vi "Periodic Tasks.vi"(8 "error in":errorcluster) -> ()   [LabVIEW 2020]
doc: "This VI runs in parallel to other tasks. It can contain as many user-defined periodic loops as you need. These can carry out PID or other sorts of timed response."
uses:
  <vilib>/Rock Robotics/WPI/ThirdParty/Sensors/navX/_TypeDefs/FRIC_navX_DeviceNumbersTypeDef.ctl
  <vilib>/Rock Robotics/WPI/ThirdParty/REV Robotics/REVLib/Typedef/Spark MAX Control Type.ctl
  <vilib>/Rock Robotics/WPI/ThirdParty/JAS_Junk/TrajLib/Rotation2d_CreateAngle.vi
  Robot Global Data.vi
  <vilib>/Rock Robotics/Network Tables/NT Write Boolean.vi
  <vilib>/Rock Robotics/Network Tables/NT Write Number.vi
  <vilib>/Rock Robotics/WPI/ThirdParty/Phoenix-LabVIEW/CANCoder/Get/CTRE_Phoenix_CANcoder_GetSensorData.vi
  Dawgma Programming Library/Utilities/armSetpoints.vi
  <vilib>/addons/control/pid/pid.llb/PID (DBL).vi
  <vilib>/Rock Robotics/WPI/ThirdParty/JAS_Junk/TrajLib/Trajectory_Library.lvlib
  <vilib>/addons/control/pid/NI_PID_pid.lvlib
  <vilib>/Rock Robotics/Network Tables/NT Read Boolean.vi
panel:
  out "arm position":dbl=0.11904771625995636
  out "Sensor Position":dbl=-2.8186375402583508e-06
  out "output":dbl=1.265315424634228e-06 format="%.2f"
  in  "SPOOL PID":T1={"proportional gain (Kc)"=0.44891030029999945, "integral time (Ti, min)"=0.0, "derivative time (Td, min)"=0.0} {"derivative time (Td, min)" format="%.29f"; "integral time (Ti, min)" format="%.29f"; "proportional gain (Kc)" format="%.29f"}
  out "arm output":dbl=0.02326189109385013 format="%.2f"
  in  "FeedFwd Value":dbl=0.04 format="%.2f"
  in  "ARM PID":T1={"proportional gain (Kc)"=0.14060000000000006, "integral time (Ti, min)"=0.0, "derivative time (Td, min)"=0.0} {"derivative time (Td, min)" format="%.15f"; "integral time (Ti, min)" format="%.15f"; "proportional gain (Kc)" format="%.15f"}
  out "POSE.TRANSLATION.Y":dbl=0.0014854368037226463
  out "POSE.TRANSLATION.X":dbl=0.0024920325622980453
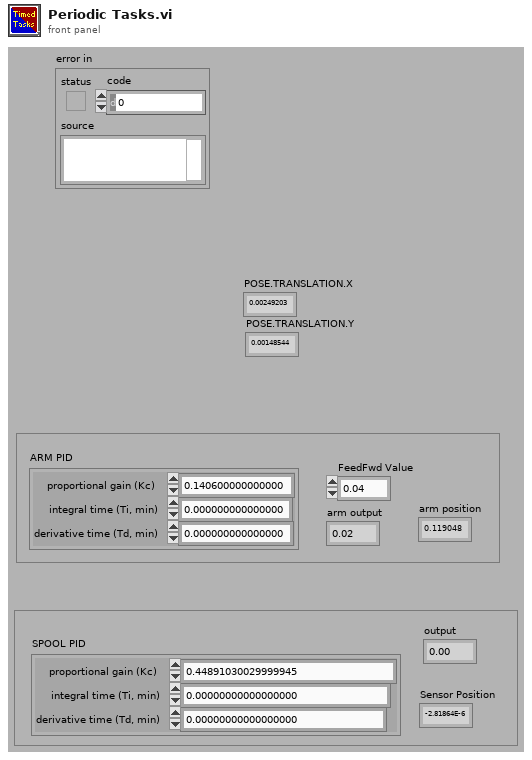
[diagram p1: front panel]
types:
  T1 = cluster{"proportional gain (Kc)":dbl, "integral time (Ti, min)":dbl, "derivative time (Td, min)":dbl}
  T2 = typedef "Trajectory_Library.lvlib/ROTATION2D.ctl" = cluster{"VALUE":dbl, "COS":dbl, "SIN":dbl}
  T3 = typedef "Trajectory_Library.lvlib/TRANSLATION2D.ctl" = cluster{"X":dbl, "Y":dbl}
  T4 = typedef "Trajectory_Library.lvlib/SWERVE_DRIVE_MODULE_POSITION.ctl" = cluster{"Distance":dbl, "Angle":T2, "P":bool}
  T5 = typedef "Trajectory_Library.lvlib/POSE2D.ctl" = cluster{"TRANSLATION":T3, "ROTATION":T2}
  T6 = typedef "Trajectory_Library.lvlib/SWERVE_DRIVE_KINEMATICS.ctl" = cluster{"NumModules":i32, "InverseKinematics":T7, "ForwardKinematics":T7, "Modules":T3[], "PrevCoR":T3, "SavedModuleStates":T8[]}
  T7 = typedef "NI_Matrix.lvlib/RealMatrix.ctl" = dbl[][]
  T8 = typedef "Trajectory_Library.lvlib/SWERVE_DRIVE_MODULE_STATE.ctl" = cluster{"Speed":dbl, "Angle":T2}
  T9 = typedef "Trajectory_Library.lvlib/SWERVE_DRIVE_ODOMETRY.ctl" = cluster{"POSE":T5, "GyroOffset":T2, "PreviousAngle":T2, "PrevModulePositions":T4[], "NumModules":i32}
  T10 = typedef "WPI_MotorControlDeviceRef.ctl" = cluster{"DeviceStatus":errorcluster, "Type":T11, "PWM":cluster{"PWM Channel":T12, "DeadBand":T13}, "CAN":cluster{"Device Number":u8, "SetOutput VI Ref":variant, "GetOutput VI Ref":variant, "Enable VI Ref":variant, "Disable VI Ref":variant, "Data":variant}, "Invert":bool, "DIO PWM":cluster{"PWM \"Enable\" Channel":T12, "DIOChannel":T14, "PWM Rate":dbl}}
  T11 = typedef "WPI_MotorControlType.ctl" = enum16{"PWM", "CAN", "DIO PWM"}
  T12 = typedef "FPGA_DIOPWMChannel.ctl" = enum8{"PWM 0", "PWM 1", "PWM 2", "PWM 3", "PWM 4", "PWM 5", "PWM 6", "PWM 7", "PWM 8", "PWM 9", "PWM MXP 0", "PWM MXP 1", "PWM MXP 2", "PWM MXP 3", "PWM MXP 4", "PWM MXP 5", "PWM MXP 6", "PWM MXP 7", "PWM MXP 8", "PWM MXP 9", "Invalid"}
  T13 = typedef "WPI_PWMDeadband.ctl" = cluster{"Name":string, "maxPositivePwm":i32, "minPositivePwm":i32, "centerPwm":i32, "maxNegativePwm":i32, "minNegativePwm":i32, "angularRange":u16}
  T14 = typedef "FPGA_DIOChannel.ctl" = enum8{"DIO 0", "DIO 1", "DIO 2", "DIO 3", "DIO 4", "DIO 5", "DIO 6", "DIO 7", "DIO 8", "DIO 9", "DIO MXP 0", "DIO MXP 1", "DIO MXP 2", "DIO MXP 3", "DIO MXP 4", "DIO MXP 5", "DIO MXP 6", "DIO MXP 7", "DIO MXP 8", "DIO MXP 9", "DIO MXP 10", "DIO MXP 11", "DIO MXP 12", "DIO MXP 13", "DIO MXP 14", "DIO MXP 15", "SPI Port CS1", "SPI Port CS2", "SPI Port CS3", "SPI Port MISO", "SPI Port MOSI", "Invalid"}
  T15 = typedef "FRIC_navX_DeviceNumbersTypeDef.ctl" = enum16{"Dev0", "Dev1", "Dev2", "Dev3"}
  T16 = cluster{"POSE.TRANSLATION.X":dbl, "POSE.TRANSLATION.Y":dbl}
  T17 = typedef "Spark MAX Control Type.ctl" = enum16{"Percent VBus", "Voltage", "Velocity", "Position", "Smart Motion", "Current", "Smart Velocity"}
  T18 = cluster{"Yaw":dbl, "Roll":dbl, "Pitch":dbl, "Heading":dbl, "Fused Heading":dbl}
  T19 = cluster{"Arm pos":dbl, "Sensor Position":dbl, "Spool pos":dbl, "Sensor Position":dbl}
  T20 = typedef "CTRE_Phoenix_CANcoder_DeviceRef.ctl" = cluster{"DeviceStatus":errorcluster, "Device Number":u8, "Handle":u64, "UsageFrame":u32, "Library Path":path}
  T21 = cluster{"FL":cluster{"proportional gain (Kc)":dbl, "integral time (Ti, min)":dbl, "derivative time (Td, min)":dbl}, "FR":cluster{"proportional gain (Kc)":dbl, "integral time (Ti, min)":dbl, "derivative time (Td, min)":dbl}, "BL":cluster{"proportional gain (Kc)":dbl, "integral time (Ti, min)":dbl, "derivative time (Td, min)":dbl}, "BR":cluster{"proportional gain (Kc)":dbl, "integral time (Ti, min)":dbl, "derivative time (Td, min)":dbl}}
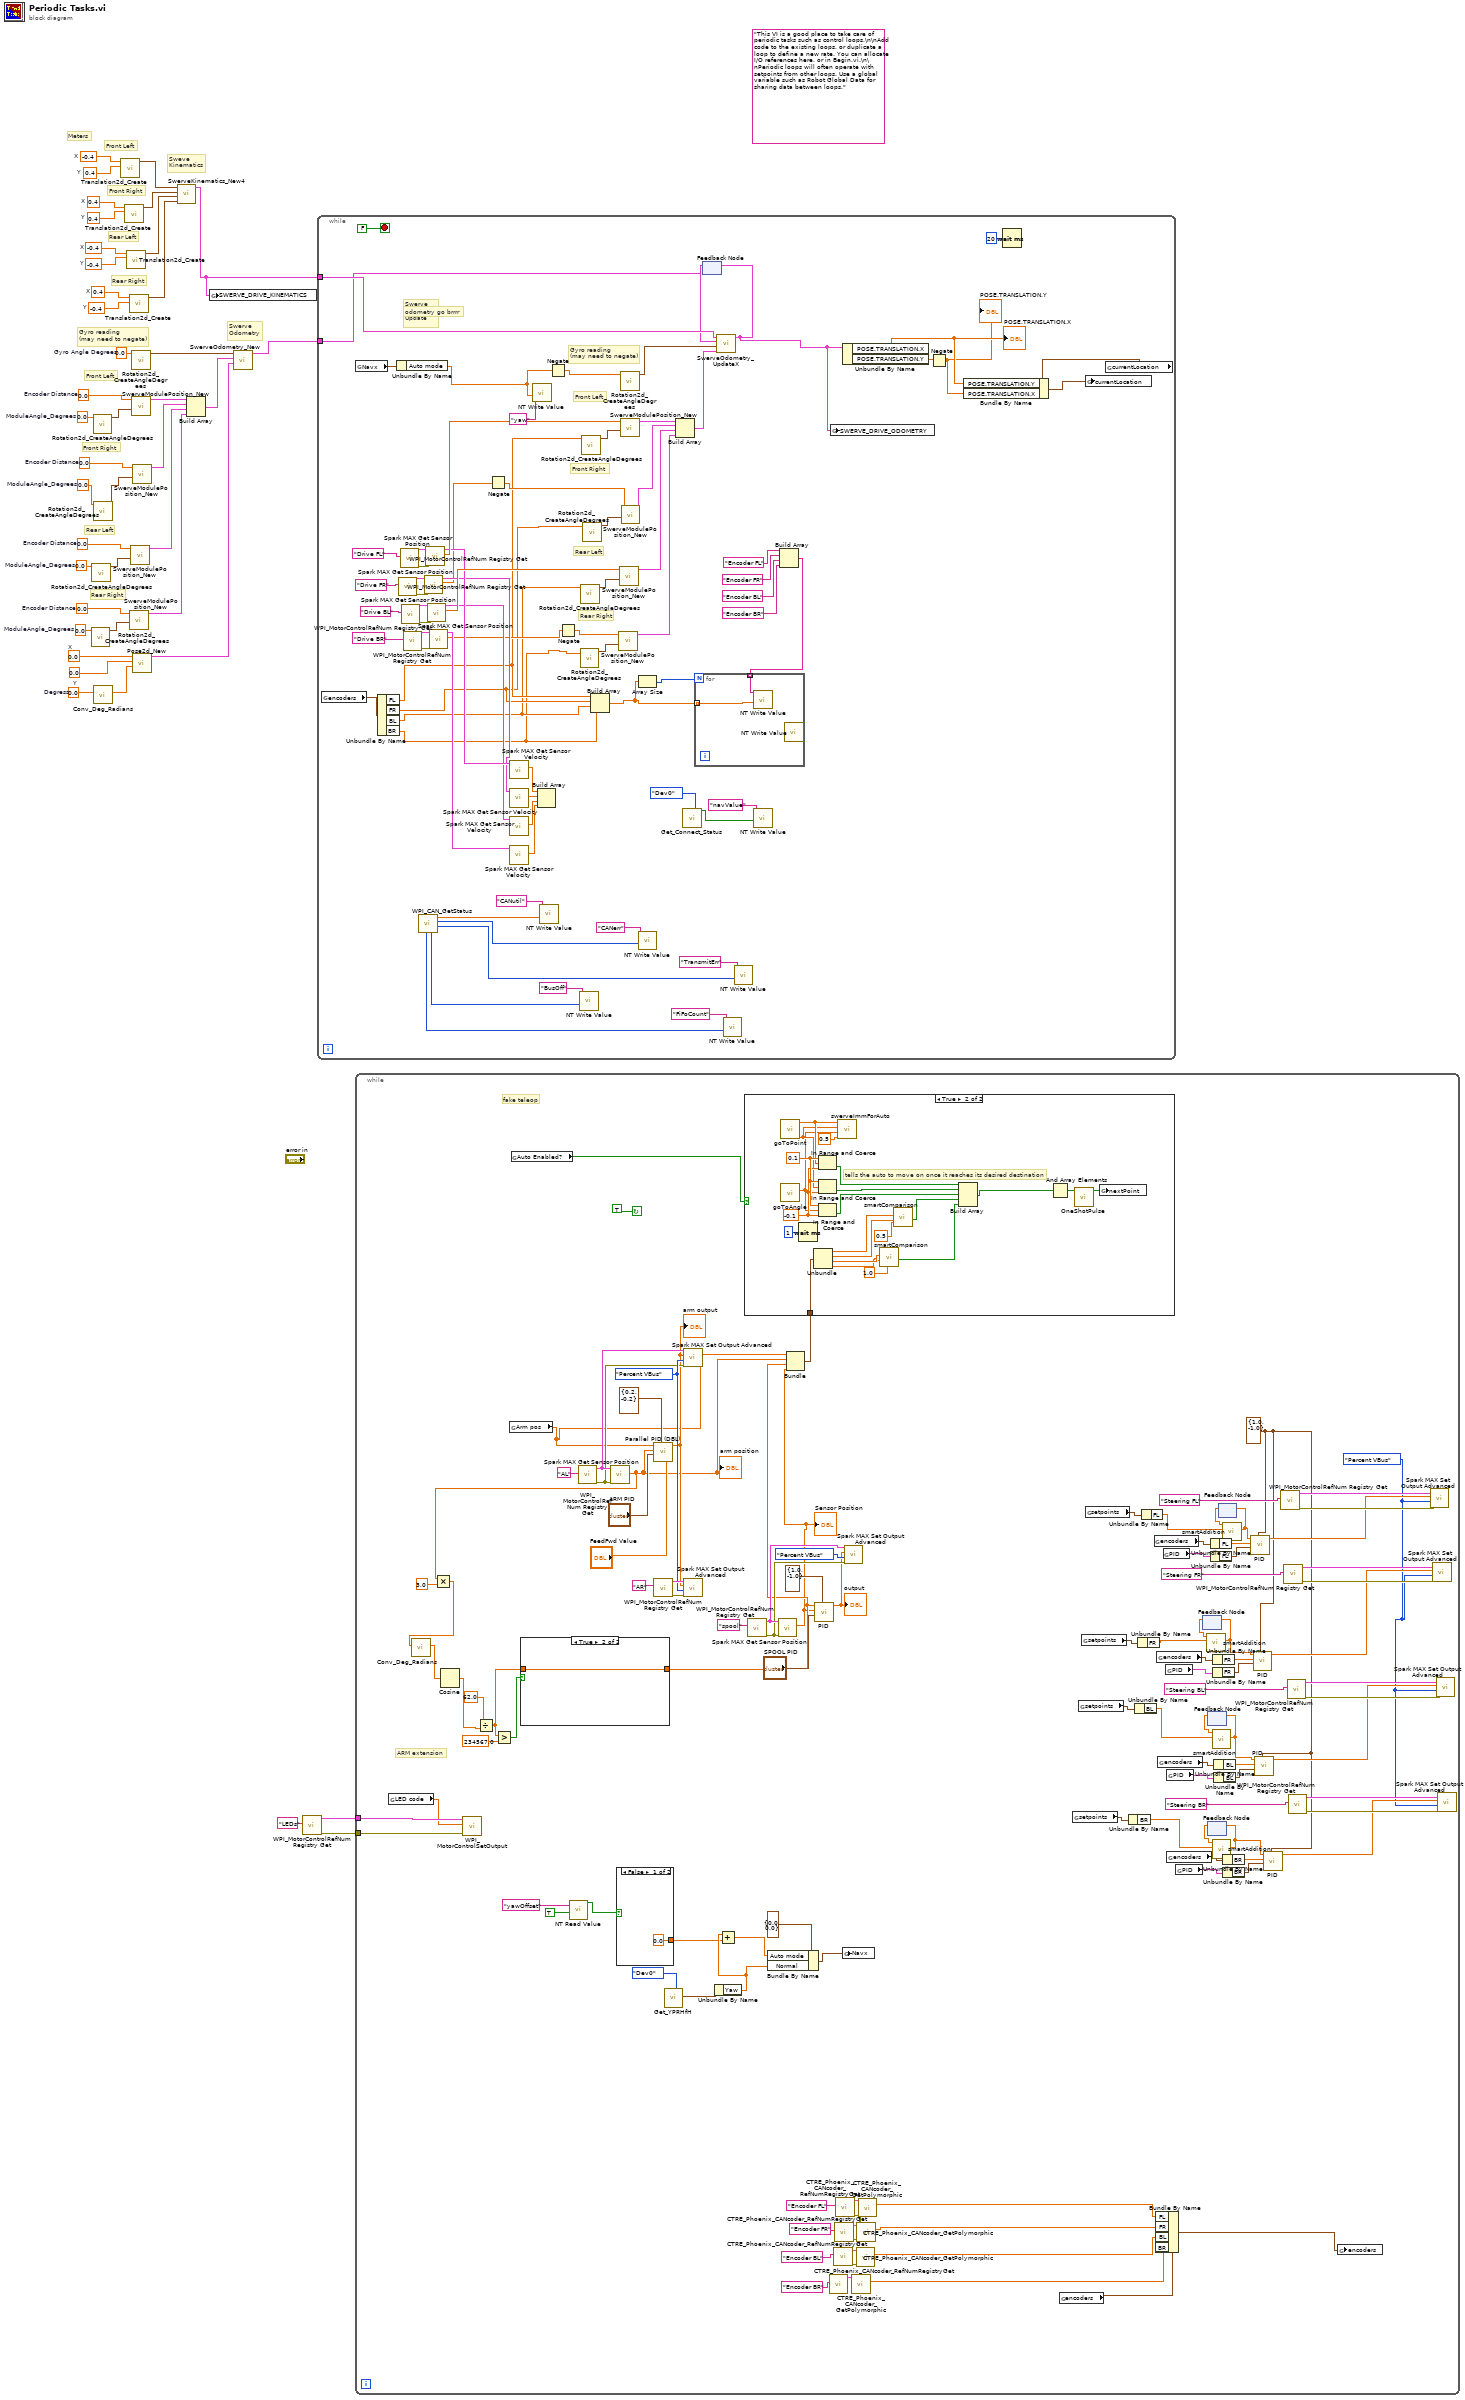
[diagram p0: block diagram]
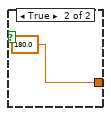
[diagram p2: hidden frame]
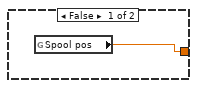
[diagram p3: hidden frame]
diagram:
  w12 = 0.4  # X
  w11 = -0.4  # Y
  w10 = -0.4  # X
  w9 = -0.4  # Y
  w8 = 0.4  # X
  w7 = 0.4  # Y
  w6 = -0.4  # X
  w5 = 0.4  # Y
  w40 = 0.0  # Degress
  w39 = 0.0  # X
  w38 = 0.0  # Y
  w31 = 0.0  # ModuleAngle_Degrees
  w29 = 0.0  # Encoder Distance
  w28 = 0.0  # ModuleAngle_Degrees
  w26 = 0.0  # Encoder Distance
  w25 = 0.0  # ModuleAngle_Degrees
  w23 = 0.0  # Encoder Distance
  w21 = 0.0  # Gyro Angle Degrees
  w20 = 0.0  # ModuleAngle_Degrees
  w18 = 0.0  # Encoder Distance
  (unwired) "This VI is a good place to take care of periodic tasks such as control loops.\n\nAdd code to the existing loops, or duplicate a loop to define a new rate. You can allocate I/O references here, or in Begin.vi.\n\nPeriodic loops will often operate with setpoints from other loops. Use a global variable such as Robot Global Data for sharing data between loops."
  # "Meters"
  # "Sweve\nKinematics"
  # "Rear Right"
  # "Rear Left"
  # "Front Right"
  # "Front Left"
  # "Swerve\nOdometry"
  # "Rear Right"
  # "Rear Left"
  # "Front Right"
  # "Front Left"
  # "Gyro reading\n(may need to negate)"
  n1 = call <vilib>:"Rotation2d_CreateAngleDegrees.vi"("Angle_Degrees"=w31) -> ("ROTATION"=w30:T2)  [unwired: 10 in]
  n2 = call <vilib>:"Rotation2d_CreateAngleDegrees.vi"("Angle_Degrees"=w28) -> ("ROTATION"=w27:T2)  [unwired: 10 in]
  n3 = call <vilib>:"Rotation2d_CreateAngleDegrees.vi"("Angle_Degrees"=w20) -> ("ROTATION"=w19:T2)  [unwired: 10 in]
  n4 = call <vilib>:"Rotation2d_CreateAngleDegrees.vi"("Angle_Degrees"=w25) -> ("ROTATION"=w24:T2)  [unwired: 10 in]
  n5 = call <vilib>:"Conv_Deg_Radians.vi"("Degress"=w40) -> ("Radians"=w37:dbl)  [unwired: 10 in]
  n6 = call <vilib>:"Translation2d_Create.vi"("Y"=w5, "X"=w6) -> ("TRANSLATION"=w13:T3)  [unwired: 9 in]
  n7 = call <vilib>:"Translation2d_Create.vi"("Y"=w7, "X"=w8) -> ("TRANSLATION"=w14:T3)  [unwired: 9 in]
  n8 = call <vilib>:"Translation2d_Create.vi"("Y"=w9, "X"=w10) -> ("TRANSLATION"=w15:T3)  [unwired: 9 in]
  n9 = call <vilib>:"Translation2d_Create.vi"("Y"=w11, "X"=w12) -> ("TRANSLATION"=w16:T3)  [unwired: 9 in]
  n10 = call <vilib>:"SwerveModulePosition_New.vi"("ROTATION"=w30, "Distance"=w29) -> ("SWERVE_DRIVE_MODULE_POSITION"=w34:T4)  [unwired: 9 in]
  n11 = call <vilib>:"SwerveModulePosition_New.vi"("ROTATION"=w27, "Distance"=w26) -> ("SWERVE_DRIVE_MODULE_POSITION"=w33:T4)  [unwired: 9 in]
  n12 = call <vilib>:"Rotation2d_CreateAngleDegrees.vi"("Angle_Degrees"=w21) -> ("ROTATION"=w35:T2)  [unwired: 10 in]
  n13 = call <vilib>:"SwerveModulePosition_New.vi"("ROTATION"=w19, "Distance"=w18) -> ("SWERVE_DRIVE_MODULE_POSITION"=w22:T4)  [unwired: 9 in]
  n14 = call <vilib>:"SwerveModulePosition_New.vi"("ROTATION"=w24, "Distance"=w23) -> ("SWERVE_DRIVE_MODULE_POSITION"=w32:T4)  [unwired: 9 in]
  n15 = call <vilib>:"Pose2d_New.vi"("Heading"=w37, "Y"=w38, "X"=w39) -> ("out POSe"=w41:T5)  [unwired: 8 in]
  n16 = call <vilib>:"SwerveKinematics_New4.vi"("wheel 3"=w16, "wheel 2"=w15, "wheel 1"=w14, "wheel 0"=w13) -> ("SWERVE_DRIVE_KINEMATICS"=w4:T6)  [unwired: 7 in]
  n17 = Build Array(w22, w32, w33, w34) -> (w36:T4[])
  n18 = global write "Robot Global Data.vi" "SWERVE_DRIVE_KINEMATICS"(w4) -> ()
  n19 = call <vilib>:"SwerveOdometry_New.vi"("InitialPose"=w41, "Module Positions"=w36, "gyroAngle"=w35) -> ("SWERVE_DRIVE_ODOMETRY"=w17:T9)  [unwired: 8 in]
  n20 = call <vilib>:"WPI_MotorControlRefNum Registry Get.vi"("refnum name"="LEDs") -> ("error out"=w1:errorcluster, "MotorControlDevRef"=w2:T10)  [unwired: 9 in]
  n21 = while {
    tunnel: w17 -> [w79]
    tunnel: w4 -> [w89]
    stop <- FALSE stop-if-true
    # "Swerve\nOdometry\nUpdate"
    # "Rear Right"
    # "Rear Left"
    # "Front Right"
    # "Front Left"
    # "Gyro reading\n(may need to negate)"
    # "odometry go brrrr"
    n22 = global read "Robot Global Data.vi" "encoders"() -> (w48:cluster{"FL":dbl, "FR":dbl, "BL":dbl, "BR":dbl})
    n23 = global read "Robot Global Data.vi" "Navx"() -> (w43:cluster{"Auto mode":dbl, "Normal":dbl})
    n24 = Unbundle By Name(w48) -> ("FL"=w47:dbl, "FR"=w46:dbl, "BL"=w45:dbl, "BR"=w44:dbl)
    n25 = Unbundle By Name(w43) -> ("Auto mode"=w42:dbl)
    n26 = call <vilib>:"WPI_MotorControlRefNum Registry Get.vi"("refnum name"="Drive FR") -> ("error out"=w105:errorcluster, "MotorControlDevRef"=w104:T10)  [unwired: 9 in]
    n27 = call <vilib>:"WPI_MotorControlRefNum Registry Get.vi"("refnum name"="Drive FL") -> ("error out"=w107:errorcluster, "MotorControlDevRef"=w106:T10)  [unwired: 9 in]
    n28 = call <vilib>:"WPI_MotorControlRefNum Registry Get.vi"("refnum name"="Drive BL") -> ("error out"=w103:errorcluster, "MotorControlDevRef"=w102:T10)  [unwired: 9 in]
    n29 = call <vilib>:"WPI_MotorControlRefNum Registry Get.vi"("refnum name"="Drive BR") -> ("error out"=w101:errorcluster, "MotorControlDevRef"=w100:T10)  [unwired: 9 in]
    n30 = call <vilib>:"WPI_CAN_GetStatus.vi"() -> ("Transmit Error Count"=w53:u32, "Receive Error Count"=w55:u32, "Percent Bus Utilization"=w58:sgl, "Bus Off Count"=w51:u32, "Transmit FIFO Full Count"=w49:u32)  [unwired: 6 in, 1 out]
    n31 = call <vilib>:"Spark MAX Get Sensor Position.vi"("error in (no error)"=w105, "MotorControlDevRef in"=w104) -> ("Sensor Position"=w75:dbl, "MotorControlDevRef out"=w87:T10)  [unwired: 6 in, 2 out]
    n32 = call <vilib>:"Spark MAX Get Sensor Position.vi"("error in (no error)"=w107, "MotorControlDevRef in"=w106) -> ("Sensor Position"=w92:dbl, "MotorControlDevRef out"=w88:T10)  [unwired: 6 in, 2 out]
    n33 = call <vilib>:"Spark MAX Get Sensor Position.vi"("error in (no error)"=w103, "MotorControlDevRef in"=w102) -> ("Sensor Position"=w91:dbl, "MotorControlDevRef out"=w86:T10)  [unwired: 6 in, 2 out]
    n34 = call <vilib>:"Spark MAX Get Sensor Position.vi"("error in (no error)"=w101, "MotorControlDevRef in"=w100) -> ("Sensor Position"=w73:dbl, "MotorControlDevRef out"=w85:T10)  [unwired: 6 in, 2 out]
    n35 = Negate(x=w75) -> (-x=w74:dbl)
    n36 = call <vilib>:"Spark MAX Get Sensor Velocity.vi"("MotorControlDevRef in"=w88) -> ("Sensor Velocity"=w84:dbl)  [unwired: 7 in, 3 out]
    n37 = call <vilib>:"Spark MAX Get Sensor Velocity.vi"("MotorControlDevRef in"=w87) -> ("Sensor Velocity"=w83:dbl)  [unwired: 7 in, 3 out]
    n38 = call <vilib>:"Spark MAX Get Sensor Velocity.vi"("MotorControlDevRef in"=w86) -> ("Sensor Velocity"=w82:dbl)  [unwired: 7 in, 3 out]
    n39 = call <vilib>:"Spark MAX Get Sensor Velocity.vi"("MotorControlDevRef in"=w85) -> ("Sensor Velocity"=w81:dbl)  [unwired: 7 in, 3 out]
    n40 = call-poly <vilib>:"NT Write Value.vi"("value"=w42, "name"="yaw") -> ()  [unwired: 9 in, 1 out]
    n41 = Build Array(w84, w83, w82, w81) -> ()  [unwired: 1 out]
    n42 = call-poly <vilib>:"NT Write Value.vi"("value"=w58, "name"="CANutil") -> ()  [unwired: 9 in, 1 out]
    n43 = Negate(x=w42) -> (-x=w76:dbl)
    n44 = Negate(x=w73) -> (-x=w72:dbl)
    n45 = call-poly <vilib>:"NT Write Value.vi"("value"=w51, "name"="BusOff") -> ()  [unwired: 9 in, 1 out]
    n46 = call <vilib>:"Rotation2d_CreateAngleDegrees.vi"("Angle_Degrees"=w44) -> ("ROTATION"=w112:T2)  [unwired: 10 in]
    n47 = call <vilib>:"Rotation2d_CreateAngleDegrees.vi"("Angle_Degrees"=w45) -> ("ROTATION"=w111:T2)  [unwired: 10 in]
    n48 = call <vilib>:"Rotation2d_CreateAngleDegrees.vi"("Angle_Degrees"=w47) -> ("ROTATION"=w108:T2)  [unwired: 10 in]
    n49 = call <vilib>:"Rotation2d_CreateAngleDegrees.vi"("Angle_Degrees"=w46) -> ("ROTATION"=w110:T2)  [unwired: 10 in]
    n50 = Build Array(w47, w46, w45, w44) -> (w68:dbl[])
    n51 = call <vilib>:"SwerveModulePosition_New.vi"("ROTATION"=w112, "Distance"=w72) -> ("SWERVE_DRIVE_MODULE_POSITION"=w115:T4)  [unwired: 9 in]
    n52 = call <vilib>:"SwerveModulePosition_New.vi"("ROTATION"=w111, "Distance"=w91) -> ("SWERVE_DRIVE_MODULE_POSITION"=w114:T4)  [unwired: 9 in]
    n53 = call <vilib>:"Rotation2d_CreateAngleDegrees.vi"("Angle_Degrees"=w76) -> ("ROTATION"=w77:T2)  [unwired: 10 in]
    n54 = call <vilib>:"SwerveModulePosition_New.vi"("ROTATION"=w108, "Distance"=w92) -> ("SWERVE_DRIVE_MODULE_POSITION"=w109:T4)  [unwired: 9 in]
    n55 = call <vilib>:"SwerveModulePosition_New.vi"("ROTATION"=w110, "Distance"=w74) -> ("SWERVE_DRIVE_MODULE_POSITION"=w113:T4)  [unwired: 9 in]
    n56 = Array Size(array=w68) -> (size(s)=w69:i32)
    n57 = call-poly <vilib>:"NT Write Value.vi"("value"=w55, "name"="CANerr") -> ()  [unwired: 9 in, 1 out]
    n58 = Build Array(w109, w113, w114, w115) -> (w95:T4[])
    n59 = call <vilib>:"Get_Connect_Status.vi"("Device Number"=FRIC_navX_DeviceNumbersTypeDef."Dev0") -> ("Connected"=w62:bool)  [unwired: 10 in]
    n60 = feedback #1(w79) -> (w80:T9)
    n61 = call <vilib>:"SwerveOdometry_UpdateX.vi"("module Positions"=w95, "gyroAngle"=w77, "in SWERVE_DRIVE_ODOMETRY"=w80, "SWERVE_DRIVE_KINEMATICS"=w89) -> ("out SWERVE_DRIVE_ODOMETRY"=w78:T9)  [unwired: 5 in, 2 out]
    n62 = feedback-in #1(w78) -> ()
    n63 = call-poly <vilib>:"NT Write Value.vi"("value"=w49, "name"="FiFoCount") -> ()  [unwired: 9 in, 1 out]
    n64 = call-poly <vilib>:"NT Write Value.vi"("value"=w53, "name"="TransmitErr") -> ()  [unwired: 9 in, 1 out]
    n65 = call-poly <vilib>:"NT Write Value.vi"("value"=w62, "name"="navValue") -> ()  [unwired: 9 in, 1 out]
    n66 = Build Array("Encoder FL", "Encoder FR", "Encoder BL", "Encoder BR") -> (w63:string[])
    n67 = for {
      N: w69 -> [_]
      tunnel: w68 -> [w119] mode=indexing
      tunnel: w63 -> [w118] mode=indexing
      n68 = call-poly <vilib>:"NT Write Value.vi"("value"=w119, "name"=w118) -> ()  [unwired: 9 in, 1 out]
    }
    n69 = global write "Robot Global Data.vi" "SWERVE_DRIVE_ODOMETRY"(w78) -> ()
    n70 = Unbundle By Name(w78) -> ("POSE.TRANSLATION.X"=w90:dbl, "POSE.TRANSLATION.Y"=w71:dbl)
    "POSE.TRANSLATION.X" <- w90
    n71 = Negate(x=w71) -> (-x=w70:dbl)
    "POSE.TRANSLATION.Y" <- w70
    n72 = Wait (ms)(milliseconds to wait=u32 20) -> ()  [unwired: 1 out]
    n73 = global read "Robot Global Data.vi" "currentLocation"() -> (w93:T16)
    n74 = Bundle By Name(cluster=w93, "POSE.TRANSLATION.Y"=w90, "POSE.TRANSLATION.X"=w70) -> (w94:T16)
    n75 = global write "Robot Global Data.vi" "currentLocation"(w94) -> ()
  }
  n76 = while {
    tunnel: w2 -> [w122]
    tunnel: w1 -> [w121]
    stop <- TRUE continue-if-true
    w159 = Spark_MAX_Control_Type."Percent VBus" ("Control Mode")
    w164 = cluster{"output high":dbl, "output low":dbl} {"output high"=1.0, "output low"=-1.0} ("output range")
    w177 = Spark_MAX_Control_Type."Percent VBus" ("Control Mode")
    # "ARM extension"
    # "fake teleop"
    n77 = global read "Robot Global Data.vi" "LED code"() -> (w120:dbl)
    n78 = call <vilib>:"WPI_MotorControlSetOutput.vi"("error in (no error)"=w121, "Output"=w120, "MotorControlDevRef"=w122) -> ()  [unwired: 6 in, 3 out]
    n79 = global read "armSetpoints.vi" "Arm pos"() -> (w145:dbl)
    n80 = global read "Robot Global Data.vi" "Auto Enabled?"() -> (w231:bool)
    n81 = call-poly <vilib>:"NT Read Value.vi"("default value"=TRUE, "name"="yawOffset") -> ("value"=w124:bool)  [unwired: 7 in, 2 out]
    n82 = call <vilib>:"WPI_MotorControlRefNum Registry Get.vi"("refnum name"="AL") -> ("error out"=w154:errorcluster, "MotorControlDevRef"=w155:T10)  [unwired: 9 in]
    n83 = call <vilib>:"Spark MAX Get Sensor Position.vi"("error in (no error)"=w154, "MotorControlDevRef in"=w155) -> ("Sensor Position"=w134:dbl)  [unwired: 6 in, 3 out]
    "arm position" <- w134
    n84 = Multiply(x=w134, y=3.0) -> (x*y=w128:dbl)
    n85 = call <vilib>:"Conv_Deg_Radians.vi"("Degress"=w128) -> ("Radians"=w127:dbl)  [unwired: 10 in]
    n86 = Cosine(x=w127) -> (cos(x)=w130:dbl)
    n87 = Divide(x=62.0 ("y"), y=w130) -> (x/y=w131:dbl)
    n88 = Greater?(x=w131, y=234567.0) -> (0:w132:bool)
    n89 = case shown="True" w132 {
      tunnel: [w235 w236] -> w144
      tunnel: w131 -> [_ w236]
      frame False {
        n90 = global read "armSetpoints.vi" "Spool pos"() -> (w235:dbl)
      }
      frame True {
      }
    }
    n91 = case shown="False" w124 {
      tunnel: [0.0 ("y") 180.0 ("y")] -> w125
      frame False {
      }
      frame True {
      }
    }
    n92 = call <vilib>:"Parallel PID (DBL).vi"("FeedFwd Value"="FeedFwd Value", "output range"=cluster{"output high":dbl, "output low":dbl} {"output high"=0.2, "output low"=-0.2}, "PID gains"="ARM PID", "process variable"=w134, "setpoint"=w145) -> ("output"=w146:dbl)  [unwired: 3 in, 3 out]
    "arm output" <- w146
    n93 = call <vilib>:"WPI_MotorControlRefNum Registry Get.vi"("refnum name"="AR") -> ("error out"=w160:errorcluster, "MotorControlDevRef"=w161:T10)  [unwired: 9 in]
    n94 = call <vilib>:"Get_YPRHfH.vi"("Device Number"=FRIC_navX_DeviceNumbersTypeDef."Dev0") -> ("YRPHfH"=w138:T18)  [unwired: 10 in]
    n95 = call <vilib>:"Spark MAX Set Output Advanced.vi"("error in (no error)"=w154, "Control Mode"=w159, "Setpoint"=w146, "MotorControlDevRef"=w155) -> ()  [unwired: 6 in, 2 out]
    n96 = call <vilib>:"Spark MAX Set Output Advanced.vi"("error in (no error)"=w160, "Control Mode"=w159, "Setpoint"=w146, "MotorControlDevRef"=w161) -> ()  [unwired: 6 in, 2 out]
    n97 = Unbundle By Name(w138) -> ("Yaw"=w137:dbl)
    n98 = Add(x=w137, y=w125) -> (x+y=w136:dbl)
    n99 = call <vilib>:"WPI_MotorControlRefNum Registry Get.vi"("refnum name"="spool") -> ("error out"=w150:errorcluster, "MotorControlDevRef"=w151:T10)  [unwired: 9 in]
    n100 = Bundle By Name(cluster=cluster{"Auto mode":dbl, "Normal":dbl} {"Auto mode"=0.0, "Normal"=0.0} ("Navx"), "Auto mode"=w136, "Normal"=w137) -> (w139:cluster{"Auto mode":dbl, "Normal":dbl})
    n101 = call <vilib>:"Spark MAX Get Sensor Position.vi"("error in (no error)"=w150, "MotorControlDevRef in"=w151) -> ("Sensor Position"=w143:dbl)  [unwired: 6 in, 3 out]
    "Sensor Position" <- w143
    n102 = Bundle("Arm pos"=w145, "Sensor Position"=w134, "Spool pos"=w144, "Sensor Position"=w143) -> (w142:T19)  [unwired: 1 in]
    n103 = case shown="True" w231 {
      tunnel: w142 -> [_ w242]
      frame False {
      }
      frame True {
        w255 = -0.1 ("lower limit")
        w256 = 0.1 ("upper limit")
        # "tells the auto to move on once it reaches its desired destination"
        n104 = call "goToPoint.vi"() -> ("y result"=w253:dbl, "x result"=w254:dbl)  [unwired: 10 in]
        n105 = call "goToAngle.vi"() -> ("x2"=w252:dbl)  [unwired: 11 in]
        n106 = Wait (ms)(milliseconds to wait=u32 1) -> ()  [unwired: 1 out]
        n107 = Unbundle(w242) -> ("Arm pos"=w241:dbl, "Sensor Position"=w240:dbl, "Spool pos"=w239:dbl, "Sensor Position"=w238:dbl)
        n108 = In Range and Coerce(upper limit=w256, x=w254, lower limit=w255) -> (In Range?=w251:bool)  [unwired: 1 out]
        n109 = In Range and Coerce(upper limit=w256, x=w253, lower limit=w255) -> (In Range?=w250:bool)  [unwired: 1 out]
        n110 = In Range and Coerce(upper limit=w256, x=w252, lower limit=w255) -> (In Range?=w249:bool)  [unwired: 1 out]
        n111 = call "swerveImmForAuto.vi"("scalespeed"=0.5 ("ScaleSpeed"), "x2"=w252, "y1"=w253, "x1"=w254) -> ()  [unwired: 8 in]
        n112 = call "smartComparison.vi"("whoCares? index"=1.0, "Process variable"=w238, "Setpoint"=w239) -> ("Happy"=w243:bool)  [unwired: 8 in]
        n113 = call "smartComparison.vi"("whoCares? index"=0.5, "Process variable"=w240, "Setpoint"=w241) -> ("Happy"=w244:bool)  [unwired: 8 in]
        n114 = Build Array(w251, w250, w249, w244, w243) -> (w248:bool[])
        n115 = And Array Elements(Boolean array=w248) -> (logical AND=w247:bool)
        n116 = call "OneShotPulse.vi"("Input"=w247) -> ("Output"=w246:bool)  [unwired: 10 in]
        n117 = global write "Robot Global Data.vi" "nextPoint"(w246) -> ()
      }
    }
    n118 = call-poly <vilib>:"PID.vi"("output range"=cluster{"output high":dbl, "output low":dbl} {"output high"=1.0, "output low"=-1.0}, "PID gains"="SPOOL PID", "process variable"=w143, "setpoint"=w144) -> ("output"=w147:dbl)  [unwired: 6 in, 1 out]
    "output" <- w147
    n119 = call <vilib>:"CTRE_Phoenix_CANcoder_RefNumRegistryGet.vi"("refnum name"="Encoder BR") -> ("CTRE_CANcoder_DeviceRef"=w224:T20)  [unwired: 9 in, 1 out]
    n120 = call <vilib>:"CTRE_Phoenix_CANcoder_RefNumRegistryGet.vi"("refnum name"="Encoder BL") -> ("error out"=w225:errorcluster, "CTRE_CANcoder_DeviceRef"=w226:T20)  [unwired: 9 in]
    n121 = call <vilib>:"CTRE_Phoenix_CANcoder_RefNumRegistryGet.vi"("refnum name"="Encoder FR") -> ("error out"=w227:errorcluster, "CTRE_CANcoder_DeviceRef"=w228:T20)  [unwired: 9 in]
    n122 = call <vilib>:"CTRE_Phoenix_CANcoder_RefNumRegistryGet.vi"("refnum name"="Encoder FL") -> ("error out"=w229:errorcluster, "CTRE_CANcoder_DeviceRef"=w230:T20)  [unwired: 9 in]
    n123 = global write "Robot Global Data.vi" "Navx"(w139) -> ()
    n124 = call <vilib>:"Spark MAX Set Output Advanced.vi"("error in (no error)"=w150, "Control Mode"=Spark_MAX_Control_Type."Percent VBus", "Setpoint"=w147, "MotorControlDevRef"=w151) -> ()  [unwired: 6 in, 2 out]
    n125 = call-poly <vilib>:"CTRE_Phoenix_CANcoder_GetPolymorphic.vi"("CTRE_CANcoder_DeviceRef"=w224) -> ("Position"=w214:dbl)  [unwired: 10 in, 4 out]
    n126 = call-poly <vilib>:"CTRE_Phoenix_CANcoder_GetPolymorphic.vi"("CTRE_CANcoder_DeviceRef"=w226, "error in"=w225) -> ("Position"=w215:dbl)  [unwired: 9 in, 4 out]
    n127 = call-poly <vilib>:"CTRE_Phoenix_CANcoder_GetPolymorphic.vi"("CTRE_CANcoder_DeviceRef"=w228, "error in"=w227) -> ("Position"=w216:dbl)  [unwired: 9 in, 4 out]
    n128 = call-poly <vilib>:"CTRE_Phoenix_CANcoder_GetPolymorphic.vi"("CTRE_CANcoder_DeviceRef"=w230, "error in"=w229) -> ("Position"=w217:dbl)  [unwired: 9 in, 4 out]
    n129 = global read "Robot Global Data.vi" "encoders"() -> (w219:cluster{"FL":dbl, "FR":dbl, "BL":dbl, "BR":dbl})
    n130 = global read "Robot Global Data.vi" "setpoints"() -> (w179:cluster{"FL":dbl, "FR":dbl, "BL":dbl, "BR":dbl})
    n131 = global read "Robot Global Data.vi" "setpoints"() -> (w188:cluster{"FL":dbl, "FR":dbl, "BL":dbl, "BR":dbl})
    n132 = global read "Robot Global Data.vi" "setpoints"() -> (w197:cluster{"FL":dbl, "FR":dbl, "BL":dbl, "BR":dbl})
    n133 = global read "Robot Global Data.vi" "setpoints"() -> (w206:cluster{"FL":dbl, "FR":dbl, "BL":dbl, "BR":dbl})
    n134 = Unbundle By Name(w179) -> ("BR"=w165:dbl)
    n135 = Unbundle By Name(w188) -> ("BL"=w168:dbl)
    n136 = Unbundle By Name(w197) -> ("FR"=w171:dbl)
    n137 = Unbundle By Name(w206) -> ("FL"=w175:dbl)
    n138 = global read "Robot Global Data.vi" "encoders"() -> (w210:cluster{"FL":dbl, "FR":dbl, "BL":dbl, "BR":dbl})
    n139 = Bundle By Name(cluster=w219, "FL"=w217, "FR"=w216, "BL"=w215, "BR"=w214) -> (w218:cluster{"FL":dbl, "FR":dbl, "BL":dbl, "BR":dbl})
    n140 = global read "Robot Global Data.vi" "encoders"() -> (w201:cluster{"FL":dbl, "FR":dbl, "BL":dbl, "BR":dbl})
    n141 = global read "Robot Global Data.vi" "encoders"() -> (w192:cluster{"FL":dbl, "FR":dbl, "BL":dbl, "BR":dbl})
    n142 = global read "Robot Global Data.vi" "PID"() -> (w208:T21)
    n143 = global read "Robot Global Data.vi" "PID"() -> (w199:T21)
    n144 = global read "Robot Global Data.vi" "PID"() -> (w190:T21)
    n145 = global read "Robot Global Data.vi" "encoders"() -> (w183:cluster{"FL":dbl, "FR":dbl, "BL":dbl, "BR":dbl})
    n146 = global read "Robot Global Data.vi" "PID"() -> (w181:T21)
    n147 = feedback #2() -> (w173:dbl)  [unwired: 1 in]
    n148 = call "smartAddition.vi"("x"=w171, "old x"=w173) -> ("y"=w172:dbl)  [unwired: 9 in]
    n149 = feedback-in #2(w172) -> ()
    n150 = feedback #3() -> (w170:dbl)  [unwired: 1 in]
    n151 = feedback #4() -> (w167:dbl)  [unwired: 1 in]
    n152 = Unbundle By Name(w210) -> ("FL"=w209:dbl)
    n153 = Unbundle By Name(w208) -> ("FL"=w207:T1)
    n154 = call "smartAddition.vi"("x"=w168, "old x"=w170) -> ("y"=w169:dbl)  [unwired: 9 in]
    n155 = feedback-in #3(w169) -> ()
    n156 = call "smartAddition.vi"("x"=w165, "old x"=w167) -> ("y"=w166:dbl)  [unwired: 9 in]
    n157 = feedback-in #4(w166) -> ()
    n158 = Unbundle By Name(w201) -> ("FR"=w200:dbl)
    n159 = Unbundle By Name(w199) -> ("FR"=w198:T1)
    n160 = Unbundle By Name(w192) -> ("BL"=w191:dbl)
    n161 = Unbundle By Name(w190) -> ("BL"=w189:T1)
    n162 = feedback #5() -> (w176:dbl)  [unwired: 1 in]
    n163 = call "smartAddition.vi"("x"=w175, "old x"=w176) -> ("y"=w174:dbl)  [unwired: 9 in]
    n164 = feedback-in #5(w174) -> ()
    n165 = Unbundle By Name(w183) -> ("BR"=w182:dbl)
    n166 = Unbundle By Name(w181) -> ("BR"=w180:T1)
    n167 = call-poly <vilib>:"PID.vi"("output range"=w164, "PID gains"=w207, "process variable"=w209, "setpoint"=w174) -> ("output"=w205:dbl)  [unwired: 6 in, 1 out]
    n168 = call-poly <vilib>:"PID.vi"("output range"=w164, "PID gains"=w198, "process variable"=w200, "setpoint"=w172) -> ("output"=w196:dbl)  [unwired: 6 in, 1 out]
    n169 = call-poly <vilib>:"PID.vi"("output range"=w164, "PID gains"=w189, "process variable"=w191, "setpoint"=w169) -> ("output"=w187:dbl)  [unwired: 6 in, 1 out]
    n170 = call-poly <vilib>:"PID.vi"("output range"=w164, "PID gains"=w180, "process variable"=w182, "setpoint"=w166) -> ("output"=w178:dbl)  [unwired: 6 in, 1 out]
    n171 = call <vilib>:"WPI_MotorControlRefNum Registry Get.vi"("refnum name"="Steering FL") -> ("error out"=w211:errorcluster, "MotorControlDevRef"=w212:T10)  [unwired: 9 in]
    n172 = call <vilib>:"WPI_MotorControlRefNum Registry Get.vi"("refnum name"="Steering FR") -> ("error out"=w202:errorcluster, "MotorControlDevRef"=w203:T10)  [unwired: 9 in]
    n173 = call <vilib>:"WPI_MotorControlRefNum Registry Get.vi"("refnum name"="Steering BL") -> ("error out"=w193:errorcluster, "MotorControlDevRef"=w194:T10)  [unwired: 9 in]
    n174 = call <vilib>:"WPI_MotorControlRefNum Registry Get.vi"("refnum name"="Steering BR") -> ("error out"=w184:errorcluster, "MotorControlDevRef"=w185:T10)  [unwired: 9 in]
    n175 = global write "Robot Global Data.vi" "encoders"(w218) -> ()
    n176 = call <vilib>:"Spark MAX Set Output Advanced.vi"("error in (no error)"=w211, "Control Mode"=w177, "Setpoint"=w205, "MotorControlDevRef"=w212) -> ()  [unwired: 6 in, 2 out]
    n177 = call <vilib>:"Spark MAX Set Output Advanced.vi"("error in (no error)"=w202, "Control Mode"=w177, "Setpoint"=w196, "MotorControlDevRef"=w203) -> ()  [unwired: 6 in, 2 out]
    n178 = call <vilib>:"Spark MAX Set Output Advanced.vi"("error in (no error)"=w193, "Control Mode"=w177, "Setpoint"=w187, "MotorControlDevRef"=w194) -> ()  [unwired: 6 in, 2 out]
    n179 = call <vilib>:"Spark MAX Set Output Advanced.vi"("error in (no error)"=w184, "Control Mode"=w177, "Setpoint"=w178, "MotorControlDevRef"=w185) -> ()  [unwired: 6 in, 2 out]
  }
  n180 = call-poly <vilib>:"NT Write Value.vi"() -> ()  [unwired: 11 in, 1 out]
